vi "Manual Assembly DB.vi"() -> ()   [LabVIEW 2021]
uses:
  Classes/Routine/Routine Enum.ctl
  Classes/Assembly/Database Entry/Database Entry.lvclass
  Classes/Assembly/Assembly Run.lvclass
  Classes/Workspace/Fixture Enum.ctl
  <vilib>/Utility/file.llb/Read Delimited Spreadsheet (string).vi
  SubVIs/PUT_region.vi
  SubVIs/component_tray_region.vi
  SubVIs/assembly_tray_region.vi
  Classes/Controller/I-O/I-O.lvclass
  Classes/Routine/Routine.lvclass
  Classes/Workspace/Fixture.lvclass
  Classes/Controller/Controller.lvclass
panel:
  out "Dummy assembly":bool
  in  "Do old-style single-module data-entry?":bool
  in  "Update comments":bool
  out "Status":string
  out "Stack names":T1
  out "Feet check":bool
  out "Assembly Type":string
  out "Assembly tray region":dbl
  out "Component tray region":dbl
  out "PUT Region":dbl
  in  "Clear All":bool
  in  "Assemble":bool
  in  "Pick and Place":bool
  in  "Dispense glue":bool
  in  "Go":bool
  in  "Routine":T2=enum."Dispense Epoxy"
  in  "Update":bool
  in  "Stage":i32(listbox)=-1
  in  "Stop":bool
  in  "Remove":bool
  in  "Add":bool
  # "Click the Run arrow to start\nFill out pop-up prompts\nSelect Full Assemble\nSelect GO"
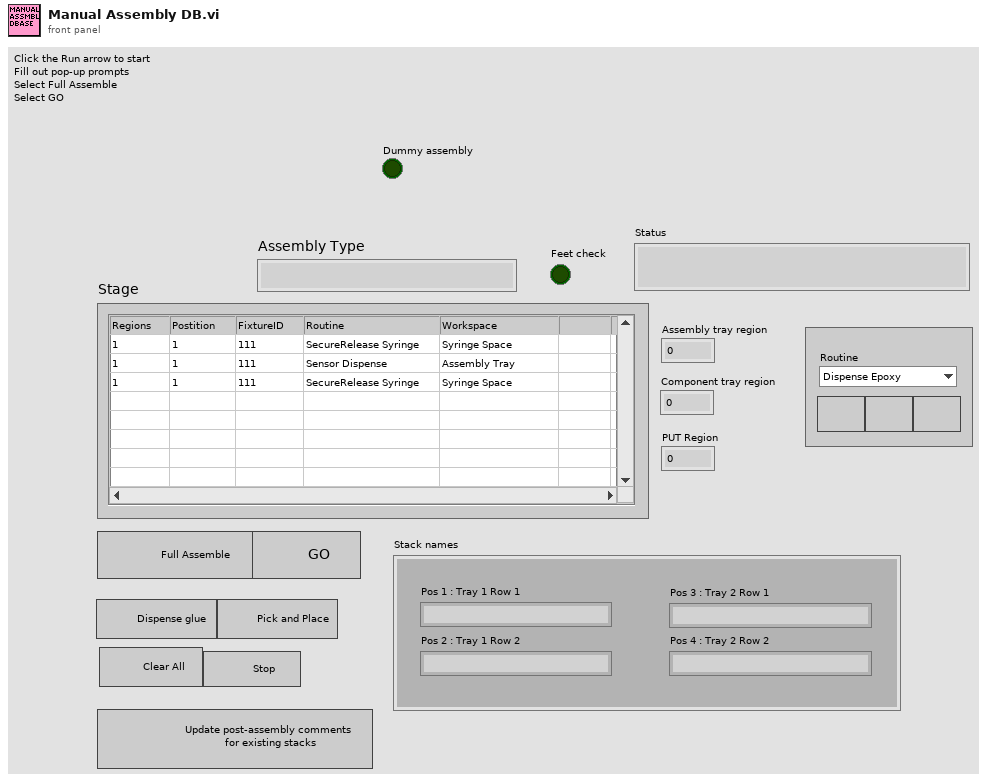
[diagram p1: front panel]
types:
  T1 = cluster{"Pos 1 : Tray 1 Row 1":string, "Pos 2 : Tray 1 Row 2":string, "Pos 3 : Tray 2 Row 1":string, "Pos 4 : Tray 2 Row 2":string}
  T2 = typedef "Routine.lvclass/Routine Enum.ctl" = enum16{"Primary Pick Up", "Secondary Pick Up", "Put Down All", "Secure Syringe", "Release Syringe", "Dispense Epoxy", "Pick Up All", "Put Down Secondary", "Full Assembly"}
  T3 = enum8{"Enabled", "Disabled", "Disabled and Grayed Out"}
  T4 = typedef "Fixture.lvclass/Fixture Enum.ctl" = enum16{"Assembly Tray", "Syringe Space", "Component", "Pick Up Tool", "Current Position"}
  T5 = cluster{"Fixture ID":dbl, "Position":dbl, "Thickness":dbl}
  T6 = typedef "File Paths.ctl" = cluster{"Glue Pattern Folder":path, "Carrier Tray Folder":path, "Pick Up Tool Fixture Folder":path, "Components Folder":path, "Bellows Tool Offset.txt":path, "Pick Up Tool Offset.txt":path, "Dispense Tip Offset.txt":path, "Log Files":path, "Gantry Assembly Map.txt":path, "Syringe and offset map.txt":path, "Controllers Folder":path, "Local dbase config":path}
  T7 = typedef "Controller.lvclass/Controllers.ctl" = cluster{"I-O.lvclass":refnum<class "I-O.lvclass">, "Gantry":refnum<k24>, "Dispenser":refnum<visa-resource-name>}
  T8 = cluster{"Fixture ID":dbl, "Position":dbl, "Thickness":dbl}[]
  T9 = cluster{"Stack names[0]":string, "Stack names[1]":string, "Stack names[2]":string, "Stack names[3]":string}
  T10 = cluster{"Fixture ID":dbl, "Position":dbl, "Thickness":dbl}[][]
  T11 = typedef "I-O.lvclass/Pin Map.ctl" = cluster{"Region Valves":i32[], "Extra Valves":dbl[][][], "Tool Primary Valve":i32, "Tool Secondary Valve":i32, "Region Sensors":i32[], "Extra Sensors":dbl[][][], "Tool Primary Sensor":dbl, "Tool Secondary Sensor":dbl, "Compression Sensor":dbl, "5V":i32, "Dispenser Sensor":dbl, "Light Curtain":i32}
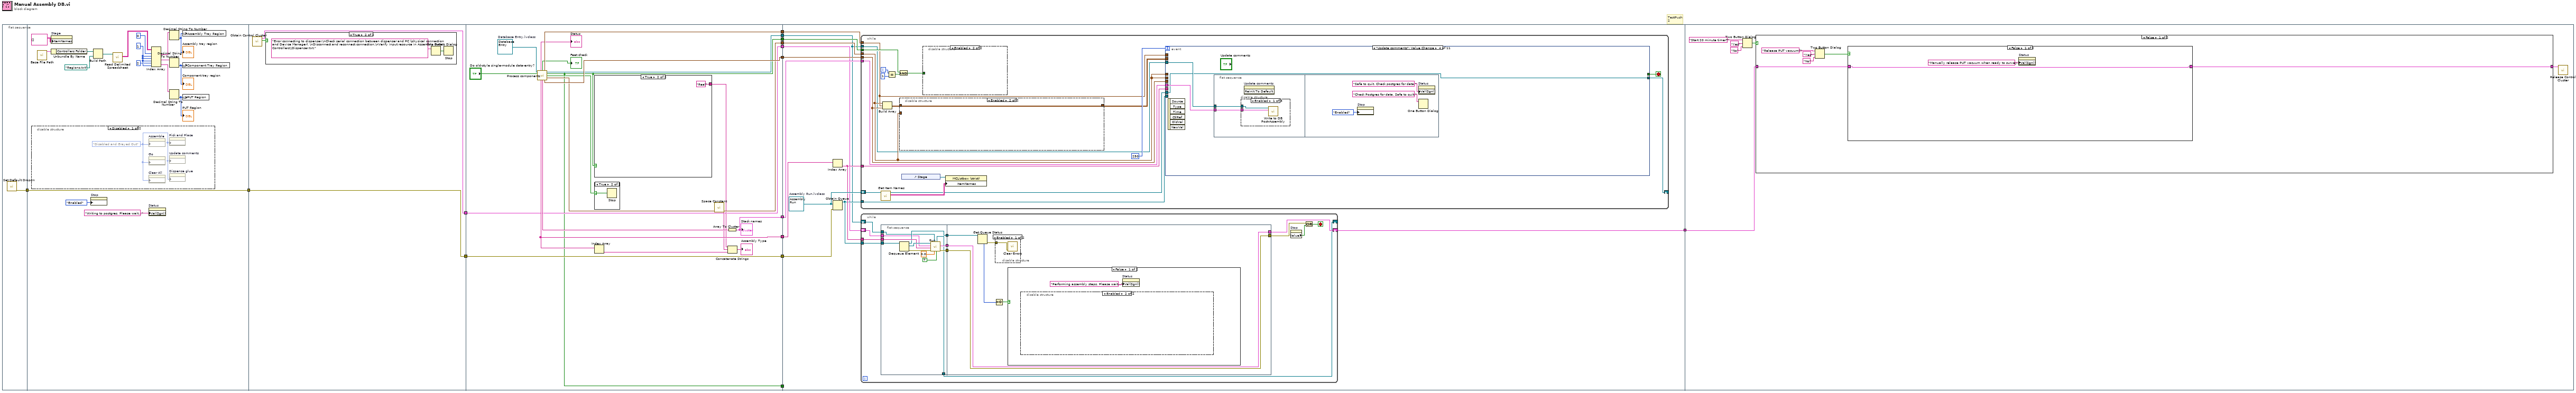
[diagram p0: block diagram]
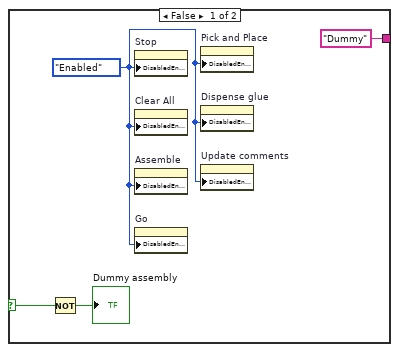
[diagram p4: hidden frame]
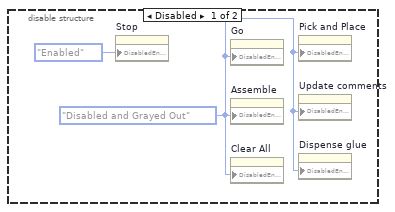
[diagram p7: hidden frame]
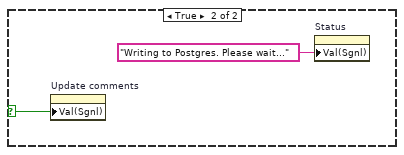
[diagram p8: hidden frame]
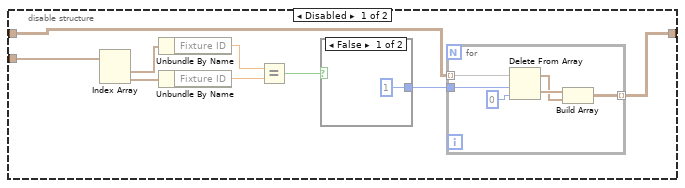
[diagram p9: hidden frame]
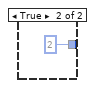
[diagram p10: hidden frame]
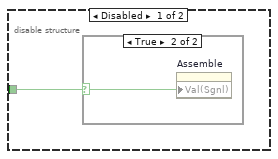
[diagram p11: hidden frame]
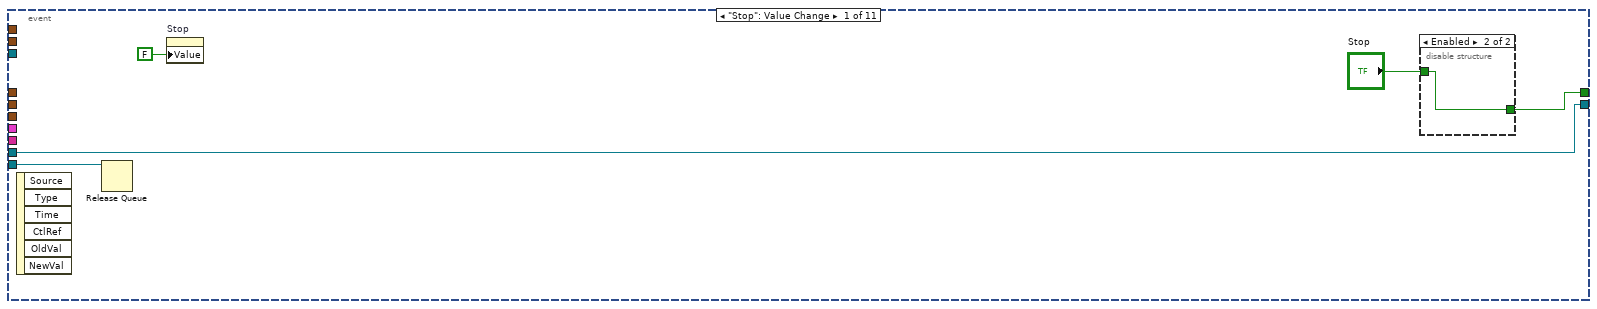
[diagram p13: hidden frame]
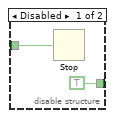
[diagram p14: hidden frame]
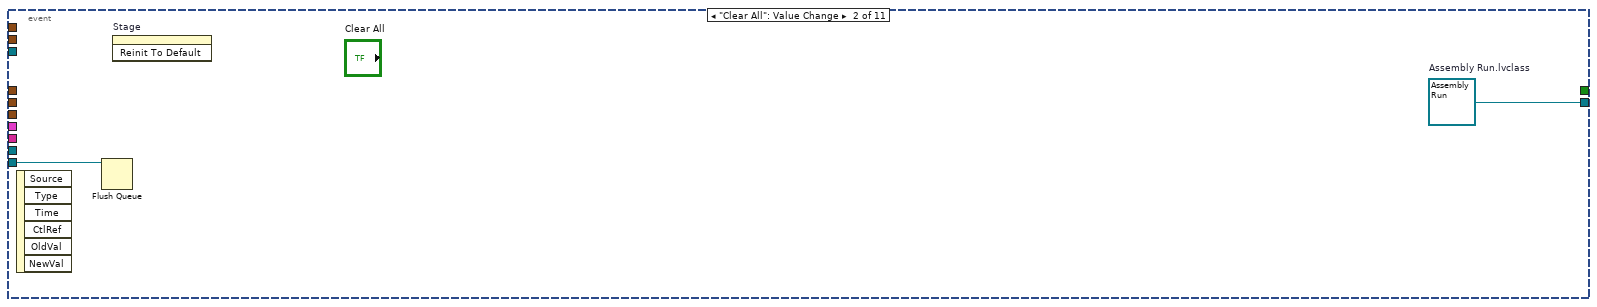
[diagram p15: hidden frame]
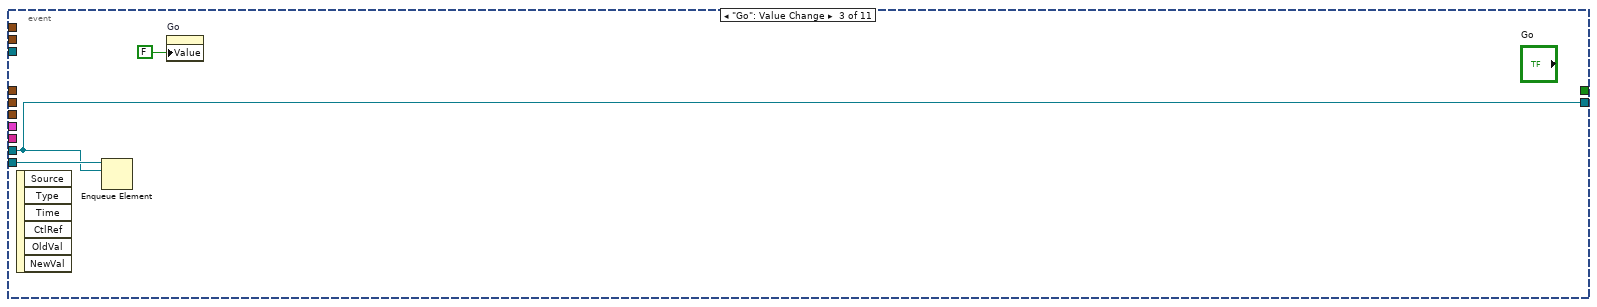
[diagram p16: hidden frame]
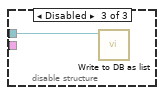
[diagram p18: hidden frame]
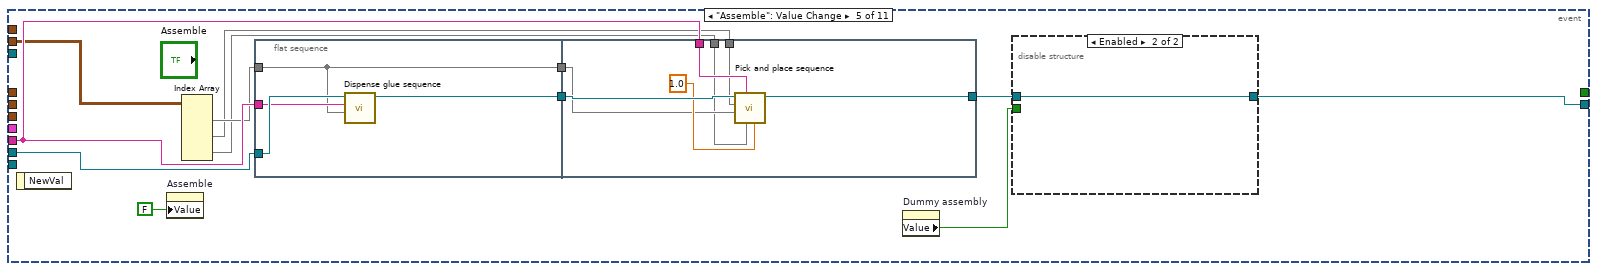
[diagram p19: hidden frame]
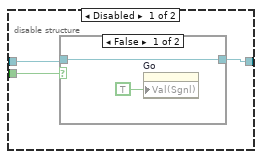
[diagram p20: hidden frame]
diagram:
  # "TestPush\n2"
  n1 = flat-sequence {
    tunnel: [w16] -> w14
    tunnel: [w20] -> w7
    tunnel: w14 -> [w20]
    tunnel: w7 -> [w38]
    tunnel: [w38] -> w6
    tunnel: [w36] -> w4
    tunnel: [w58] -> w15
    tunnel: w6 -> [w58]
    tunnel: [w57] -> w13
    tunnel: [w56] -> w12
    tunnel: [w55] -> w11
    tunnel: [w47] -> w10
    tunnel: [w51] -> w9
    tunnel: [w49] -> w8
    tunnel: [w42] -> w5
    tunnel: w4 -> [w42]
    tunnel: [w41] -> w3
    tunnel: [w41] -> w2
    tunnel: w15 -> [w77]
    tunnel: w13 -> [w76]
    tunnel: w12 -> [w75]
    tunnel: w11 -> [w70]
    tunnel: w10 -> [w74]
    tunnel: w9 -> [w72]
    tunnel: w8 -> [w66]
    tunnel: w5 -> [w69]
    tunnel: w3 -> [w68]
    tunnel: w2 -> [_]
    tunnel: [w67] -> w1
    tunnel: w1 -> [w374]
    frame #0 {
      n2 = call "Set Default Drop-In.vi"() -> ("error out"=w16:errorcluster)  [unwired: 11 in]
    }
    frame #1 {
      w23 = 1 ("disabled index (col)")
      n3 = disable-structure shown="Disabled" {
        frame Disabled {
          w35 = T3."Disabled and Grayed Out" ("Disabled")
          n4 = property on="Assemble" class="Bool (strict)"("DisabledEnum"=w35) -> ()  [unwired: 2 in, 2 out]
          n5 = property on="Go" class="Bool (strict)"("DisabledEnum"=w35) -> ()  [unwired: 2 in, 2 out]
          n6 = property on="Clear All" class="Bool"("DisabledEnum"=w35) -> ()  [unwired: 2 in, 2 out]
          n7 = property on="Pick and Place" class="Bool"("DisabledEnum"=w35) -> ()  [unwired: 2 in, 2 out]
          n8 = property on="Update comments" class="Bool (strict)"("DisabledEnum"=w35) -> ()  [unwired: 2 in, 2 out]
          n9 = property on="Dispense glue" class="Bool"("DisabledEnum"=w35) -> ()  [unwired: 2 in, 2 out]
        }
        frame Enabled {
        }
      }
      n10 = call "Base File Path.vi"() -> ("Paths Out"=w34:T6)  [unwired: 11 in]
      n11 = property on="Stage" class="MCListbox (strict)"("ItemNames"=string[][] []) -> ()  [unwired: 2 in, 2 out]
      n12 = Unbundle By Name(w34) -> ("Controllers Folder"=w32:path)
      n13 = property on="Stop" class="Bool (strict)"("DisabledEnum"=T3."Enabled" ("Disabled")) -> ()  [unwired: 2 in, 2 out]
      n14 = Build Path(base path=w32, name or relative path=path "Regions.txt") -> (appended path=w33:path)
      n15 = call-poly <vilib>:"Read Delimited Spreadsheet.vi"("file path (dialog if empty)"=w33) -> ("all rows"=w21:string[][])  [unwired: 9 in, 5 out]
      n16 = property on="Status" class="Str"("Val(Sgnl)"="Writing to postgres. Please wait..." ("Value (Signaling)")) -> ()  [unwired: 2 in, 2 out]
      n17 = Index Array(array=w21, index (row) #1=0 ("index (row)"), index (col) #1=w23, index (row) #2=w23, index (col) #2=w23, index (row) #3=2 ("disabled index (row)"), index (col) #3=w23) -> (element #1=w26:string, element #2=w25:string, element #3=w27:string)
      n18 = Decimal String To Number(string=w26) -> (number=w29:i32)  [unwired: 2 in, 1 out]
      "Assembly tray region" <- w29
      n19 = Decimal String To Number(string=w25) -> (number=w30:i32)  [unwired: 2 in, 1 out]
      "Component tray region" <- w30
      n20 = Decimal String To Number(string=w27) -> (number=w28:i32)  [unwired: 2 in, 1 out]
      "PUT Region" <- w28
      n21 = global write "assembly_tray_region.vi" "Assembly Tray Region"(w29) -> ()
      n22 = global write "component_tray_region.vi" "Component Tray Region"(w30) -> ()
      n23 = global write "PUT_region.vi" "PUT Region"(w28) -> ()
    }
    frame #2 {
      n24 = call "Obtain Control Cluster.vi"() -> ("Dispenser error?"=w37:bool, "Control Out"=w36:T7)  [unwired: 10 in]
      n25 = case shown="True" w37 {
        frame False {
        }
        frame True {
          n26 = One Button Dialog(message="Error connecting to dispenser.\nCheck serial connection between dispenser and PC (physical connection and Device Manager). \nDisconnect and reconnect connection.\nVerify input resource in Assembly Data\\Controllers\\Dispenser.txt.") -> (true=w39:bool)  [unwired: 1 in]
          n27 = Stop(stop? (T)=w39) -> ()
        }
      }
    }
    frame #3 {
      w59 = refnum<class "Database Entry.lvclass"> refnum  # Database Entry.lvclass
      n28 = call "Process components.vi"("Database Entry in"=w59, "Do single-module data entry?"="Do old-style single-module data-entry?") -> ("Status"=→"Status":string, "Feet check"=→"Feet check":bool, "PUT Settings"=w56:T8, "Database Entry out"=w49:refnum<class "Database Entry.lvclass">, "Is real run?"=w41:bool, "Aborted"=w52:bool, "Assembly Settings"=w55:T8, "Assembly Type"=w47:string[], "Stack names"=w54:string[], "Component Settings"=w57:T8)  [unwired: 2 in, 2 out]
      n29 = case shown="True" w41 {
        selector: w41 -> [w61 _]
        tunnel: ["Dummy" "Real"] -> w44
        frame False {
          w62 = T3."Enabled" ("Disabled")
          n30 = Not(x=w61) -> (.not. x?=→"Dummy assembly":bool)
          n31 = property on="Stop" class="Bool (strict)"("DisabledEnum"=w62) -> ()  [unwired: 2 in, 2 out]
          n32 = property on="Clear All" class="Bool"("DisabledEnum"=w62) -> ()  [unwired: 2 in, 2 out]
          n33 = property on="Assemble" class="Bool (strict)"("DisabledEnum"=w62) -> ()  [unwired: 2 in, 2 out]
          n34 = property on="Go" class="Bool (strict)"("DisabledEnum"=w62) -> ()  [unwired: 2 in, 2 out]
          n35 = property on="Pick and Place" class="Bool"("DisabledEnum"=w62) -> ()  [unwired: 2 in, 2 out]
          n36 = property on="Dispense glue" class="Bool"("DisabledEnum"=w62) -> ()  [unwired: 2 in, 2 out]
          n37 = property on="Update comments" class="Bool (strict)"("DisabledEnum"=w62) -> ()  [unwired: 2 in, 2 out]
        }
        frame True {
        }
      }
      n38 = case shown="True" w52 {
        selector: w52 -> [_ w65]
        frame False {
        }
        frame True {
          n39 = Stop(stop? (T)=w65) -> ()
        }
      }
      n40 = Index Array(array=w47) -> (element=w46:string)  [unwired: 1 in]
      n41 = call <vilib>:"Space Constant.vi"() -> ("String"=w45:string)
      n42 = Array To Cluster(array=w54) -> (cluster=w51:T9)
      "Stack names" <- w51
      n43 = Concatenate Strings(w44, w45, w46) -> (→"Assembly Type":string)
    }
    frame #4 {
      w78 = refnum<class "Assembly Run.lvclass"> refnum  # Assembly Run.lvclass
      n44 = Index Array(array=w74) -> (element=w73:string)  [unwired: 1 in]
      n45 = Obtain Queue(element data type=w78, error in (no error)=w77) -> (queue out=w71:refnum<queue>)  [unwired: 3 in, 2 out]
      n46 = while {
        shift-right: [w129] -> _
        shift-left: w78 -> [w131]
        tunnel: w71 -> [w134]
        tunnel: w73 -> [w128]
        tunnel: w66 -> [w115]
        tunnel: w72 -> [w127]
        tunnel: w75 -> [w119]
        tunnel: w70 -> [w120]
        tunnel: w76 -> [w118]
        tunnel: w68 -> [w126]
        i -> [w125]
        stop <- w135 stop-if-true
        n47 = call "Get Item Names.vi"("Assembly Run in"=w131) -> ("Item names"=w133:string[][], "Assembly Run out"=w130:refnum<class "Assembly Run.lvclass">)  [unwired: 8 in, 1 out]
        n48 = Build Array(w120, w119, w118) -> (w117:T10)
        n49 = Equal?(x=w125, y=1) -> (x = y?=w123:bool)
        n50 = And(x=w126, y=w123) -> (x .and. y?=w122:bool)
        n51 = disable-structure shown="Enabled" {
          disable-tunnel: w120 -> [w144 _]
          disable-tunnel: w117 -> [w137 w153]
          disable-tunnel: [w136 w153] -> w116
          frame Disabled {
            n52 = Index Array(array=w144) -> (element #1=w143:T5, element #2=w142:T5)  [unwired: 2 in]
            n53 = Unbundle By Name(w143) -> ("Fixture ID"=w141:dbl)
            n54 = Unbundle By Name(w142) -> ("Fixture ID"=w140:dbl)
            n55 = Equal?(x=w141, y=w140) -> (x = y?=w139:bool)
            n56 = case shown="False" w139 {
              tunnel: [1 2] -> w138
              frame False {
              }
              frame True {
              }
            }
            n57 = for {
              tunnel: w137 -> [w150] mode=indexing
              tunnel: [w149] -> w136 mode=indexing
              tunnel: w138 -> [w145]
              n58 = Delete From Array(array=w150, length=w145, index=0) -> (deleted portion=w147:T8, array with subset deleted=w146:T8)
              n59 = Build Array(w147, w146) -> (w149:T10)
            }
          }
          frame Enabled {
          }
        }
        n60 = control-ref of="Stage"() -> (w132:refnum<vi>)
        n61 = disable-structure shown="Enabled" {
          disable-tunnel: w122 -> [w154 _]
          frame Disabled {
            n62 = case shown="True" w154 {
              selector: w154 -> [_ w155]
              frame False {
              }
              frame True {
                n63 = property on="Assemble" class="Bool (strict)"("Val(Sgnl)"=w155) -> ()  [unwired: 2 in, 2 out]
              }
            }
          }
          frame Enabled {
          }
        }
        n64 = property class="MCListbox (strict)"(reference=w132, "ItemNames"=w133) -> ()  [unwired: 1 in, 2 out]
        n65 = event shown="[3] \"Update comments\": Value Change" {
          selector: _ -> [_ _ _ _ _ _ _ _ _ _ _]
          dyn-events: _ -> [_ _ _ _ _ _ _ _ _ _ _]
          timeout: 250 -> [_ _ _ _ _ _ _ _ _ _ _]
          tunnel: [w157 _ _ _ _ _ _ _ _ _ _] -> w135
          tunnel: w130 -> [w160 _ w167 w169 w191 w210 w215 w223 w233 w365 w368]
          tunnel: [w160 w165 w167 w169 w183 w210 w214 w222 w234 w364 w367] -> w129
          tunnel: w134 -> [w159 w164 w168 _ _ _ _ _ _ _ _]
          tunnel: w118 -> [_ _ _ _ _ _ _ _ _ _ _]
          tunnel: w119 -> [_ _ _ _ _ _ _ _ _ _ _]
          tunnel: w128 -> [_ _ _ _ w190 _ w213 w221 w232 w361 _]
          tunnel: w115 -> [_ _ _ w171 _ _ _ _ _ _ _]
          tunnel: w127 -> [_ _ _ w170 _ _ _ _ _ _ _]
          tunnel: w120 -> [_ _ _ _ _ _ _ _ _ _ _]
          tunnel: w120 -> [_ _ _ _ _ _ _ _ w224 w359 _]
          tunnel: w116 -> [_ _ _ _ w182 _ w212 w216 _ _ _]
          event "Stop": Value Change {
            n66 = event-data() -> ()  [unwired: 1 in, 6 out]
            n67 = Release Queue(queue=w159) -> ()  [unwired: 2 in, 3 out]
            n68 = property on="Stop" class="Bool (strict)"("Value"=FALSE ("Value (Signaling)")) -> ()  [unwired: 2 in, 2 out]
            n69 = disable-structure shown="Enabled" {
              disable-tunnel: "Stop" -> [w162 w163]
              disable-tunnel: [TRUE w163] -> w157
              frame Disabled {
                n70 = Stop(stop? (T)=w162) -> ()
              }
              frame Enabled {
              }
            }
          }
          event "Clear All": Value Change {
            w165 = refnum<class "Assembly Run.lvclass"> refnum  # Assembly Run.lvclass
            n71 = event-data() -> ()  [unwired: 1 in, 6 out]
            n72 = Flush Queue(queue=w164) -> ()  [unwired: 1 in, 3 out]
            n73 = invoke on="Stage" class="MCListbox (strict)" method="Reinit To Default"() -> ()  [unwired: 3 in, 3 out]
          }
          event "Go": Value Change {
            n74 = event-data() -> ()  [unwired: 1 in, 6 out]
            n75 = Enqueue Element(queue=w168, element=w167) -> ()  [unwired: 2 in, 3 out]
            n76 = property on="Go" class="Bool (strict)"("Value"=FALSE ("Go")) -> ()  [unwired: 2 in, 2 out]
          }
          event "Update comments": Value Change {
            n77 = event-data() -> ()  [unwired: 1 in, 6 out]
            n78 = flat-sequence {
              tunnel: w171 -> [w173]
              tunnel: w170 -> [w172]
              frame #0 {
                n79 = disable-structure shown="Enabled" {
                  disable-tunnel: w173 -> [w175 _ w176]
                  disable-tunnel: w172 -> [w174 _ _]
                  frame Enabled {
                    n80 = call "Write to DB Post-Assembly.vi"("Stack names"=w174, "Database Entry in"=w175) -> ()  [unwired: 8 in, 2 out]
                  }
                  frame Disabled {
                  }
                  frame Disabled {
                    n81 = call "Write to DB as list.vi"("Database Entry in"=w176) -> ()  [unwired: 8 in, 3 out]
                  }
                }
                n82 = invoke on="Update comments" class="Bool (strict)" method="Reinit To Default"() -> ()  [unwired: 3 in, 3 out]
              }
              frame #1 {
                n83 = property on="Stop" class="Bool (strict)"("DisabledEnum"=T3."Enabled" ("Disabled")) -> ()  [unwired: 2 in, 2 out]
                n84 = property on="Status" class="Str"("Val(Sgnl)"="Safe to quit. Check postgres for data.") -> ()  [unwired: 2 in, 2 out]
                n85 = One Button Dialog(message="Check Postgres for data. Safe to quit.") -> ()  [unwired: 1 in, 1 out]
              }
            }
          }
          event "Assemble": Value Change {
            n86 = event-data() -> ()  [unwired: 1 in, 1 out]
            n87 = property on="Assemble" class="Bool (strict)"("Value"=FALSE ("Assemble")) -> ()  [unwired: 2 in, 2 out]
            n88 = Index Array(array=w182) -> (element #1=w189:T8, element #2=w188:T8, element #3=w187:T8)  [unwired: 6 in]
            n89 = flat-sequence {
              tunnel: [w194] -> w181
              tunnel: w191 -> [w195]
              tunnel: w190 -> [w193]
              tunnel: w189 -> [w192]
              tunnel: [w192] -> w180
              tunnel: [w201] -> w184
              tunnel: w181 -> [w202]
              tunnel: w190 -> [w200]
              tunnel: w180 -> [w198]
              tunnel: w188 -> [w197]
              tunnel: w187 -> [w196]
              frame #0 {
                n90 = call "Dispense glue sequence.vi"("Assembly Tray Settings Array"=w192, "Assembly Type"=w193, "Assembly Run in"=w195) -> ("Assembly Run out"=w194:refnum<class "Assembly Run.lvclass">)  [unwired: 7 in, 1 out]
              }
              frame #1 {
                n91 = call "Pick and place sequence.vi"("Numeric"=1.0, "Component Tray map"=w196, "Assembly Type"=w200, "Assembly Tray map"=w198, "PUT map"=w197, "Assembly Run in"=w202) -> ("Assembly Run out"=w201:refnum<class "Assembly Run.lvclass">)  [unwired: 4 in, 1 out]
              }
            }
            n92 = property on="Dummy assembly" class="Bool (strict)"() -> ("Value"=w185:bool)  [unwired: 2 in, 2 out]
            n93 = disable-structure shown="Enabled" {
              disable-tunnel: w185 -> [w205 _]
              disable-tunnel: w184 -> [w204 w209]
              disable-tunnel: [w203 w209] -> w183
              frame Disabled {
                n94 = case shown="False" w205 {
                  tunnel: w204 -> [w207 w208]
                  tunnel: [w207 w208] -> w203
                  frame False {
                    n95 = property on="Go" class="Bool (strict)"("Val(Sgnl)"=TRUE ("Value (Signaling)")) -> ()  [unwired: 2 in, 2 out]
                  }
                  frame True {
                  }
                }
              }
              frame Enabled {
              }
            }
          }
          event Timeout {
            n96 = event-data() -> ()  [unwired: 1 in, 3 out]
          }
          event "Dispense glue": Value Change {
            n97 = event-data() -> ()  [unwired: 1 in, 1 out]
            n98 = Index Array(array=w212) -> (element=w211:T8)  [unwired: 2 in]
            n99 = call "Dispense glue sequence.vi"("Assembly Tray Settings Array"=w211, "Assembly Type"=w213, "Assembly Run in"=w215) -> ("Assembly Run out"=w214:refnum<class "Assembly Run.lvclass">)  [unwired: 7 in, 1 out]
          }
          event "Pick and Place": Value Change {
            n100 = event-data() -> ()  [unwired: 1 in, 6 out]
            n101 = Index Array(array=w216) -> (element #1=w219:T8, element #2=w218:T8, element #3=w217:T8)  [unwired: 6 in]
            n102 = call "Pick and place sequence.vi"("Numeric"=1.0, "Component Tray map"=w217, "Assembly Type"=w221, "Assembly Tray map"=w219, "PUT map"=w218, "Assembly Run in"=w223) -> ("Assembly Run out"=w222:refnum<class "Assembly Run.lvclass">)  [unwired: 4 in, 1 out]
          }
          event "Add": Value Change {
            n103 = event-data() -> ()  [unwired: 1 in, 1 out]
            n104 = local read "Routine"() -> (w228:T2)
            n105 = case shown="\"Primary Pick Up\"" w228 {
              tunnel: [Fixture_Enum."Assembly Tray" ("Fixture") Fixture_Enum."Pick Up Tool" ("Fixture") Fixture_Enum."Component" ("Fixture") Fixture_Enum."Assembly Tray" ("Fixture") Fixture_Enum."Assembly Tray" ("Fixture") Fixture_Enum."Assembly Tray" ("Fixture") Fixture_Enum."Syringe Space" ("Fixture") Fixture_Enum."Syringe Space" ("Fixture")] -> w231
              tunnel: w224 -> [w256 w259 w278 w297 w316 w335 w354 w357]
              tunnel: [_ w258 w279 w296 w315 w334 w353 w356] -> w225
              tunnel: [w256 _ _ _ _ _ _ _] -> w226
              frame "Dispense Epoxy", Default {
              }
              frame "Primary Pick Up" {
                n106 = call "Prompt User for Input"() -> ("Position"=w260:dbl)  [unwired: 17 in, 2 out]
                n107 = for {
                  tunnel: w260 -> [w262]
                  tunnel: w259 -> [w266] mode=indexing
                  tunnel: [w263] -> w258
                  stop <- w264 stop-if-true
                  n108 = Unbundle By Name(w266) -> ("Position"=w267:dbl)
                  n109 = Equal?(x=w267, y=w262) -> (x = y?=w265:bool)
                  n110 = case shown="False" w265 {
                    selector: w265 -> [w274 w276]
                    tunnel: w266 -> [_ w275]
                    tunnel: [w274 w276] -> w264
                    tunnel: [T5 {"Fixture ID"=0.0, "Position"=0.0, "Thickness"=0.0} ("Settings") w275] -> w263
                    tunnel: w262 -> [w269 _]
                    frame False {
                      n111 = Number To Decimal String(number=w269) -> (decimal integer string=w270:string)  [unwired: 1 in]
                      n112 = Concatenate Strings("Position " ("message"), w270, " not available." ("message")) -> (w268:string)
                      n113 = One Button Dialog(message=w268) -> ()  [unwired: 1 in, 1 out]
                    }
                    frame True {
                    }
                  }
                }
              }
              frame "Secondary Pick Up" {
                n114 = call "Prompt User for Input2"() -> ("Position"=w277:dbl)  [unwired: 17 in, 2 out]
                n115 = for {
                  tunnel: w277 -> [w281]
                  tunnel: w278 -> [w285] mode=indexing
                  tunnel: [w282] -> w279
                  stop <- w283 stop-if-true
                  n116 = Unbundle By Name(w285) -> ("Position"=w286:dbl)
                  n117 = Equal?(x=w286, y=w281) -> (x = y?=w284:bool)
                  n118 = case shown="False" w284 {
                    selector: w284 -> [w293 w295]
                    tunnel: w285 -> [_ w294]
                    tunnel: [w293 w295] -> w283
                    tunnel: [T5 {"Fixture ID"=0.0, "Position"=0.0, "Thickness"=0.0} ("Settings") w294] -> w282
                    tunnel: w281 -> [w288 _]
                    frame False {
                      n119 = Number To Decimal String(number=w288) -> (decimal integer string=w289:string)  [unwired: 1 in]
                      n120 = Concatenate Strings("Position " ("message"), w289, " not available." ("message")) -> (w287:string)
                      n121 = One Button Dialog(message=w287) -> ()  [unwired: 1 in, 1 out]
                    }
                    frame True {
                    }
                  }
                }
              }
              frame "Pick Up All" {
                n122 = call "Prompt User for Input3"() -> ("Position"=w298:dbl)  [unwired: 17 in, 2 out]
                n123 = for {
                  tunnel: w298 -> [w300]
                  tunnel: w297 -> [w304] mode=indexing
                  tunnel: [w301] -> w296
                  stop <- w302 stop-if-true
                  n124 = Unbundle By Name(w304) -> ("Position"=w305:dbl)
                  n125 = Equal?(x=w305, y=w300) -> (x = y?=w303:bool)
                  n126 = case shown="False" w303 {
                    selector: w303 -> [w312 w314]
                    tunnel: w304 -> [_ w313]
                    tunnel: [w312 w314] -> w302
                    tunnel: [T5 {"Fixture ID"=0.0, "Position"=0.0, "Thickness"=0.0} ("Settings") w313] -> w301
                    tunnel: w300 -> [w307 _]
                    frame False {
                      n127 = Number To Decimal String(number=w307) -> (decimal integer string=w308:string)  [unwired: 1 in]
                      n128 = Concatenate Strings("Position " ("message"), w308, " not available." ("message")) -> (w306:string)
                      n129 = One Button Dialog(message=w306) -> ()  [unwired: 1 in, 1 out]
                    }
                    frame True {
                    }
                  }
                }
              }
              frame "Put Down Secondary" {
                n130 = call "Prompt User for Input4"() -> ("Position"=w317:dbl)  [unwired: 17 in, 2 out]
                n131 = for {
                  tunnel: w317 -> [w319]
                  tunnel: w316 -> [w323] mode=indexing
                  tunnel: [w320] -> w315
                  stop <- w321 stop-if-true
                  n132 = Unbundle By Name(w323) -> ("Position"=w324:dbl)
                  n133 = Equal?(x=w324, y=w319) -> (x = y?=w322:bool)
                  n134 = case shown="False" w322 {
                    selector: w322 -> [w331 w333]
                    tunnel: w323 -> [_ w332]
                    tunnel: [w331 w333] -> w321
                    tunnel: [T5 {"Fixture ID"=0.0, "Position"=0.0, "Thickness"=0.0} ("Settings") w332] -> w320
                    tunnel: w319 -> [w326 _]
                    frame False {
                      n135 = Number To Decimal String(number=w326) -> (decimal integer string=w327:string)  [unwired: 1 in]
                      n136 = Concatenate Strings("Position " ("message"), w327, " not available." ("message")) -> (w325:string)
                      n137 = One Button Dialog(message=w325) -> ()  [unwired: 1 in, 1 out]
                    }
                    frame True {
                    }
                  }
                }
              }
              frame "Put Down All" {
                n138 = call "Prompt User for Input5"() -> ("Position"=w336:dbl)  [unwired: 17 in, 2 out]
                n139 = for {
                  tunnel: w336 -> [w338]
                  tunnel: w335 -> [w342] mode=indexing
                  tunnel: [w339] -> w334
                  stop <- w340 stop-if-true
                  n140 = Unbundle By Name(w342) -> ("Position"=w343:dbl)
                  n141 = Equal?(x=w343, y=w338) -> (x = y?=w341:bool)
                  n142 = case shown="False" w341 {
                    selector: w341 -> [w350 w352]
                    tunnel: w342 -> [_ w351]
                    tunnel: [w350 w352] -> w340
                    tunnel: [T5 {"Fixture ID"=0.0, "Position"=0.0, "Thickness"=0.0} ("Settings") w351] -> w339
                    tunnel: w338 -> [w345 _]
                    frame False {
                      n143 = Number To Decimal String(number=w345) -> (decimal integer string=w346:string)  [unwired: 1 in]
                      n144 = Concatenate Strings("Position " ("message"), w346, " not available." ("message")) -> (w344:string)
                      n145 = One Button Dialog(message=w344) -> ()  [unwired: 1 in, 1 out]
                    }
                    frame True {
                    }
                  }
                }
              }
              frame "Secure Syringe" {
                n146 = Index Array(array=w354) -> (element=w353:T5)  [unwired: 1 in]
              }
              frame "Release Syringe" {
                n147 = Index Array(array=w357) -> (element=w356:T5)  [unwired: 1 in]
              }
            }
            n148 = Equal?(x=w228, y=Routine_Enum."Dispense Epoxy") -> (x = y?=w229:bool)
            n149 = case shown="True" w229 {
              tunnel: [w241 w255] -> w234
              tunnel: w233 -> [w240 w254]
              tunnel: w232 -> [w239 w253]
              tunnel: w231 -> [w238 w252]
              tunnel: w228 -> [w237 w251]
              tunnel: TRUE ("Auto") -> [w236 w250]
              tunnel: w226 -> [w235 _]
              tunnel: w225 -> [_ w249]
              frame True {
                n150 = for {
                  tunnel: w239 -> [w246]
                  tunnel: w238 -> [w245]
                  tunnel: w237 -> [w244]
                  tunnel: w236 -> [w243]
                  shift-right: [w248] -> w241
                  shift-left: w240 -> [w247]
                  tunnel: w235 -> [w242] mode=indexing
                  n151 = call-dynamic "Add Single.vi"("UI in"=w247, "Routine"=w244, "Assembly Type"=w246, "Fixture"=w245, "Input Settings"=w242, "Auto"=w243) -> ("UI out"=w248:refnum<class "Assembly Run.lvclass">)  [unwired: 8 in, 1 out]
                }
              }
              frame False {
                n152 = call-dynamic "Add Single.vi"("UI in"=w254, "Routine"=w251, "Assembly Type"=w253, "Fixture"=w252, "Input Settings"=w249, "Auto"=w250) -> ("UI out"=w255:refnum<class "Assembly Run.lvclass">)  [unwired: 8 in, 1 out]
              }
            }
          }
          event "Update": Value Change {
            n153 = event-data() -> ()  [unwired: 1 in, 6 out]
            n154 = Index Array(array=w359) -> (element=w360:T5)  [unwired: 1 in]
            n155 = call "Update.vi"("Input Settings"=w360, "Assembly Type"=w361, "Row"="Stage", "Routine"="Routine", "Assembly Run in"=w365) -> ("Assembly Run out"=w364:refnum<class "Assembly Run.lvclass">)  [unwired: 5 in, 1 out]
          }
          event "Remove": Value Change {
            n156 = event-data() -> ()  [unwired: 1 in, 6 out]
            n157 = local read "Stage"() -> (w366:i32)
            n158 = call "Delete.vi"("Index"=w366, "Assembly In"=w368) -> ("Assembly Out"=w367:refnum<class "Assembly Run.lvclass">)  [unwired: 8 in, 1 out]
          }
        }
      }
      n159 = while {
        shift-right: [w90] -> w67
        shift-left: w69 -> [w79]
        tunnel: w73 -> [w89]
        tunnel: w71 -> [w88]
        shift-right: [w80] -> _
        shift-left: w66 -> [w81]
        stop <- w83 stop-if-true
        n160 = flat-sequence {
          tunnel: w89 -> [w99]
          tunnel: w88 -> [w96]
          tunnel: [w100] -> w87
          tunnel: [w98] -> w86
          tunnel: [w97] -> w85
          tunnel: w81 -> [w93]
          tunnel: [w92] -> w80
          tunnel: w79 -> [w91]
          tunnel: [w107] -> w84
          tunnel: [w108] -> w90
          tunnel: w87 -> [w108]
          tunnel: w86 -> [w107]
          tunnel: w85 -> [w106]
          frame #0 {
            n161 = Dequeue Element(queue=w96) -> (queue out=w97:refnum<queue>, element=w102:refnum<class "Assembly Run.lvclass">, error out=w101:errorcluster)  [unwired: 2 in, 1 out]
            n162 = call-dynamic "Run.vi"("Dispense?"=TRUE, "Pickup_Test_Number"=0.0, "Database Entry in"=w93, "error in (no error)"=w101, "Assembly Type"=w99, "Control In"=w91, "Assembly In"=w102) -> ("error out"=w98:errorcluster, "Control Out"=w100:T7, "Database Entry out"=w92:refnum<class "Database Entry.lvclass">)  [unwired: 1 in, 1 out]
          }
          frame #1 {
            n163 = Get Queue Status(queue=w106) -> (error out=w103:errorcluster, # elements in queue=w105:i32)  [unwired: 2 in, 6 out]
            n164 = Equal To 0?(x=w105) -> (x = 0?=w104:bool)
            n165 = disable-structure shown="Enabled" {
              disable-tunnel: w103 -> [w109 _]
              frame Enabled {
                n166 = call <vilib>:"Clear Errors.vi"("error in (no error)"=w109) -> ()  [unwired: 5 in, 2 out]
              }
              frame Disabled {
              }
            }
            n167 = case shown="False" w104 {
              selector: w104 -> [_ w114]
              frame False {
                n168 = disable-structure shown="Enabled" {
                  frame Disabled {
                    w112 = T3."Disabled and Grayed Out" ("Disabled")
                    n169 = property on="Stop" class="Bool (strict)"("DisabledEnum"=T3."Enabled" ("Disabled")) -> ()  [unwired: 2 in, 2 out]
                    n170 = property on="Go" class="Bool (strict)"("DisabledEnum"=w112) -> ()  [unwired: 2 in, 2 out]
                    n171 = property on="Assemble" class="Bool (strict)"("DisabledEnum"=w112) -> ()  [unwired: 2 in, 2 out]
                    n172 = property on="Clear All" class="Bool"("DisabledEnum"=w112) -> ()  [unwired: 2 in, 2 out]
                    n173 = property on="Pick and Place" class="Bool"("DisabledEnum"=w112) -> ()  [unwired: 2 in, 2 out]
                    n174 = property on="Update comments" class="Bool (strict)"("DisabledEnum"=w112) -> ()  [unwired: 2 in, 2 out]
                    n175 = property on="Dispense glue" class="Bool"("DisabledEnum"=w112) -> ()  [unwired: 2 in, 2 out]
                  }
                  frame Enabled {
                  }
                }
                n176 = property on="Status" class="Str"("Val(Sgnl)"="Performing assembly steps. Please wait...") -> ()  [unwired: 2 in, 2 out]
              }
              frame True {
                n177 = property on="Update comments" class="Bool (strict)"("Val(Sgnl)"=w114) -> ()  [unwired: 2 in, 2 out]
                n178 = property on="Status" class="Str"("Val(Sgnl)"="Writing to Postgres. Please wait...") -> ()  [unwired: 2 in, 2 out]
              }
            }
          }
        }
        n179 = property on="Stop" class="Bool (strict)"() -> ("Value"=w82:bool)  [unwired: 2 in, 2 out]
        n180 = Or(x=w84, y=w82) -> (x .or. y?=w83:bool)
      }
    }
    frame #5 {
      n181 = Two Button Dialog(message="Start 20 minute timer?", 1:"No" ("F button name (\"Cancel\")"), 2:"Yes" ("T button name (\"OK\")")) -> (T button?=w369:bool)
      n182 = case shown="False" w369 {
        tunnel: w374 -> [w380 w408]
        tunnel: [w379 w404] -> w373
        frame False {
          n183 = Two Button Dialog(message="Release PUT vacuum?", 1:"No" ("F button name (\"Cancel\")"), 2:"Yes" ("T button name (\"OK\")")) -> (T button?=w375:bool)
          n184 = case shown="False" w375 {
            tunnel: w380 -> [w382 w385]
            tunnel: [w382 w383] -> w379
            frame False {
              n185 = property on="Status" class="Str"("Val(Sgnl)"="Manually release PUT vacuum when ready to survey." ("Value (Signaling)")) -> ()  [unwired: 2 in, 2 out]
            }
            frame True {
              n186 = flat-sequence {
                tunnel: w385 -> [w387]
                tunnel: [w386] -> w384
                tunnel: w384 -> [w402]
                tunnel: [w402] -> w383
                frame #0 {
                  n187 = in-place {
                    n188 = in-place-cluster #1(w387) -> ("I-O.lvclass"=w389:refnum<class "I-O.lvclass">)
                    n189 = call-dynamic "Read Pin Map.vi"("I-O in"=w389) -> ("Pin Map 2"=w394:T11, "I-O out"=w391:refnum<class "I-O.lvclass">)  [unwired: 8 in, 1 out]
                    n190 = Unbundle By Name(w394) -> ("Extra Valves"=w393:dbl[][][])
                    n191 = Index Array(array=w393, index (dim 0)=0 ("index (page)")) -> (element=w392:dbl[][])  [unwired: 2 in]
                    n192 = for {
                      tunnel: w392 -> [w400] mode=indexing
                      shift-right: [w398] -> w388
                      shift-left: w391 -> [w399]
                      n193 = Index Array(array=w400, index=0) -> (element=w397:dbl)
                      n194 = call-dynamic "Digital Write 1 Channel.vi"("Value"=FALSE, "Channel"=w397, "I-O.lvclass"=w399) -> ("I-O.lvclass 2"=w398:refnum<class "I-O.lvclass">)  [unwired: 7 in, 1 out]
                    }
                    n195 = in-place-cluster #1("I-O.lvclass"=w388) -> (w386:T7)
                  }
                }
                frame #1 {
                  n196 = property on="Status" class="Str"("Val(Sgnl)"="PUT vacuum has been released." ("Value (Signaling)")) -> ()  [unwired: 2 in, 2 out]
                }
              }
            }
          }
        }
        frame True {
          n197 = flat-sequence {
            tunnel: w408 -> [w410]
            tunnel: [w409] -> w407
            tunnel: w407 -> [w432]
            tunnel: [w432] -> w406
            tunnel: [w429] -> w405
            tunnel: w406 -> [w434]
            tunnel: w405 -> [w435]
            tunnel: [w433] -> w403
            tunnel: [w458] -> w404
            tunnel: w403 -> [w458]
            frame #0 {
              n198 = while {
                shift-right: [w423] -> w409
                shift-left: w410 -> [w423]
                stop <- w427 stop-if-true
                w417 = "%#g" ("format string")
                w426 = 1200.0 ("Time Target (s)")
                n199 = call "Elapsed Time"("Time Target (s)"=w426) -> ("Elapsed Time (s)"=w425:dbl, "Time has Elapsed"=w427:bool)  [unwired: 11 in, 6 out]
                n200 = Subtract(x=w426, y=w425) -> (x-y=w422:dbl)
                n201 = Quotient & Remainder(x=w422, y=60.0) -> (x-y*floor(x/y)=w420:dbl, floor(x/y)=w419:dbl)
                n202 = Round To Nearest(number=w420) -> (nearest integer value=w412:dbl)
                n203 = Round To Nearest(number=w419) -> (nearest integer value=w411:dbl)
                n204 = Format Into String(format string=w417, initial string="PUT vacuum will release after ", w411) -> (resulting string=w414:string)  [unwired: 1 in, 1 out]
                n205 = Format Into String(format string=w417, initial string=" minutes and ", w412) -> (resulting string=w418:string)  [unwired: 1 in, 1 out]
                n206 = Concatenate Strings(w414, w418, " seconds." ("string")) -> (w421:string)
                n207 = property on="Status" class="Str"("Val(Sgnl)"=w421) -> ()  [unwired: 2 in, 2 out]
              }
            }
            frame #1 {
              n208 = Two Button Dialog(message="20 minute curing period is complete. Release PUT vacuum?", 1:"No" ("F button name (\"Cancel\")"), 2:"Yes" ("T button name (\"OK\")")) -> (T button?=w429:bool)
            }
            frame #2 {
              n209 = case shown="True" w435 {
                tunnel: w434 -> [w437 w440]
                tunnel: [w437 w438] -> w433
                frame False {
                  n210 = property on="Status" class="Str"("Val(Sgnl)"="Manually release PUT vacuum when ready to survey." ("Value (Signaling)")) -> ()  [unwired: 2 in, 2 out]
                }
                frame True {
                  n211 = flat-sequence {
                    tunnel: w440 -> [w442]
                    tunnel: [w441] -> w439
                    tunnel: w439 -> [w457]
                    tunnel: [w457] -> w438
                    frame #0 {
                      n212 = in-place {
                        n213 = in-place-cluster #2(w442) -> ("I-O.lvclass"=w444:refnum<class "I-O.lvclass">)
                        n214 = call-dynamic "Read Pin Map.vi"("I-O in"=w444) -> ("Pin Map 2"=w449:T11, "I-O out"=w446:refnum<class "I-O.lvclass">)  [unwired: 8 in, 1 out]
                        n215 = Unbundle By Name(w449) -> ("Extra Valves"=w448:dbl[][][])
                        n216 = Index Array(array=w448, index (dim 0)=0 ("index (page)")) -> (element=w447:dbl[][])  [unwired: 2 in]
                        n217 = for {
                          tunnel: w447 -> [w455] mode=indexing
                          shift-right: [w453] -> w443
                          shift-left: w446 -> [w454]
                          n218 = Index Array(array=w455, index=0) -> (element=w452:dbl)
                          n219 = call-dynamic "Digital Write 1 Channel.vi"("Value"=FALSE, "Channel"=w452, "I-O.lvclass"=w454) -> ("I-O.lvclass 2"=w453:refnum<class "I-O.lvclass">)  [unwired: 7 in, 1 out]
                        }
                        n220 = in-place-cluster #2("I-O.lvclass"=w443) -> (w441:T7)
                      }
                    }
                    frame #1 {
                      n221 = property on="Status" class="Str"("Val(Sgnl)"="PUT vacuum has been released." ("Value (Signaling)")) -> ()  [unwired: 2 in, 2 out]
                    }
                  }
                }
              }
            }
            frame #3 {
              n222 = disable-structure shown="Enabled" {
                frame Disabled {
                  n223 = property on="Stop" class="Bool (strict)"("Val(Sgnl)"=TRUE ("Value (Signaling)")) -> ()  [unwired: 2 in, 2 out]
                }
                frame Enabled {
                }
              }
            }
          }
        }
      }
      n224 = call "Release Control Cluster.vi"("output cluster"=w373) -> ()  [unwired: 11 in]
    }
  }
